vi "Exceldispatch.vi"() -> ()   [LabVIEW 2012]
uses:
  <vilib>/Utility/NIReport.llb/NI_report.lvclass
  Global1.vi
  <vilib>/addons/database/Connection.llb/DB Tools Open Connec (Path).vi
  <vilib>/addons/_office/excel.llb/Excel Get Data (str).vi
  <vilib>/Utility/NIReport.llb/Excel/NI_Excel.lvclass
  <vilib>/addons/_office/NI_ReportGenerationToolkit.lvlib
  <vilib>/addons/database/NI_Database_API.lvlib
panel:
  out "error out 4":errorcluster
  in  "start (0, 0)":cluster{"start row":i32, "start column":i32}
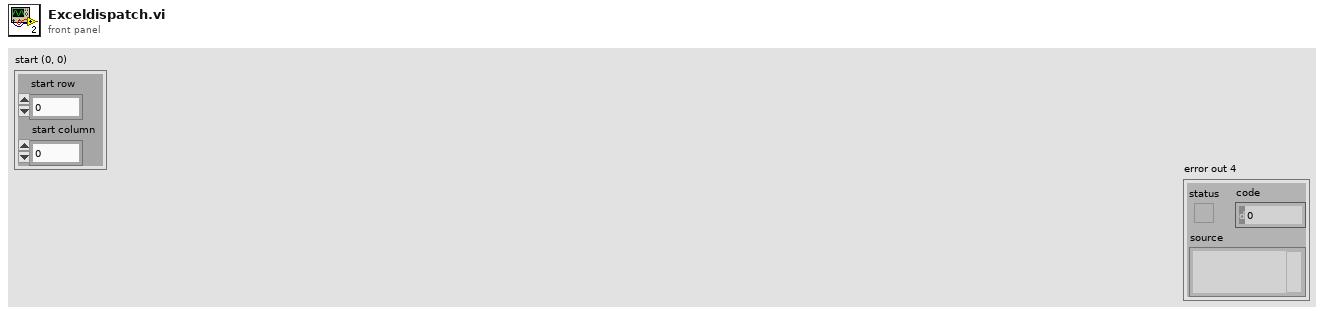
[diagram p1: front panel]
types:
  T1 = enum16{"Standard Report", "HTML", "Word", "Excel"}
  T2 = typedef "NI_Database_API.lvlib/Conn ObjectReference.ctl" = refnum<k1>
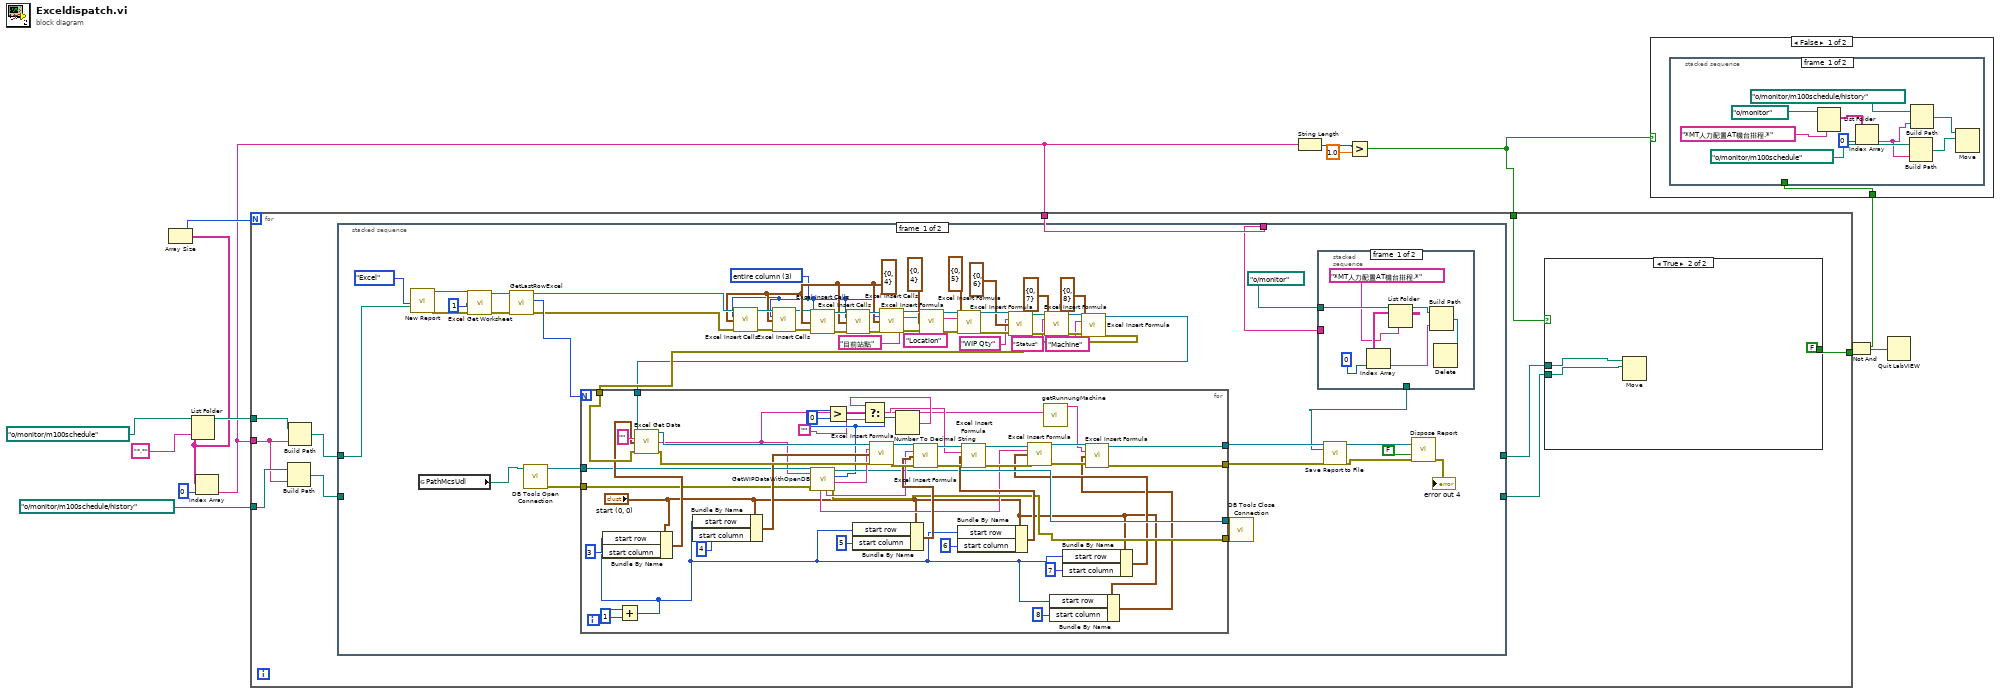
[diagram p0: block diagram]
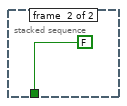
[diagram p2: hidden frame]
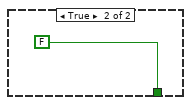
[diagram p3: hidden frame]
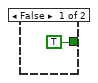
[diagram p4: hidden frame]
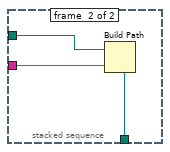
[diagram p5: hidden frame]
diagram:
  n1 = List Folder(path=path "o:/monitor/m100schedule", pattern="*.*") -> (path out=w10:path, filenames=w9:string[])  [unwired: 2 in, 2 out]
  n2 = Array Size(array=w9) -> (size(s)=w11:i32)
  n3 = Index Array(array=w9, index=0) -> (element=w3:string)
  n4 = String Length(string=w3) -> (length=w6:i32)
  n5 = Greater?(x=w6, y=1.0) -> (0:w2:bool)
  n6 = for {
    N: w11 -> [_]
    tunnel: w10 -> [w24]
    tunnel: w3 -> [w22]
    tunnel: path "o:/monitor/m100schedule/history" ("base path") -> [w23]
    tunnel: w2 -> [w17]
    tunnel: [w16] -> w4
    tunnel: w3 -> [w15]
    n7 = Build Path(base path=w23, name or relative path=w22) -> (appended path=w20:path)
    n8 = Build Path(base path=w24, name or relative path=w22) -> (appended path=w21:path)
    n9 = stacked-sequence {
      tunnel: w21 -> [w59 w141]
      tunnel: w20 -> [_ w142]
      tunnel: [_ w142] -> w18
      tunnel: [_ w141] -> w19
      tunnel: w15 -> [w30 _]
      frame #0 {
        w47 = cluster{"row":i32, "column":i32} {"row"=0, "column"=4} ("start (0, 0)")
        w44 = u16 3 items=["shift cells right", "shift cells down", "entire row", "entire column"] ("mode (entire row)")
        n10 = call <vilib>:"New Report.vi"("report type"=T1."Excel" ("Report Type"), "template (empty)"=w59) -> ("report out"=w83:refnum<class "NI_report.lvclass">, "error out"=w82:errorcluster)  [unwired: 12 in]
        n11 = global read "Global1.vi" "PathMcsUdl"() -> (w74:path)
        n12 = call <vilib>:"Excel Get Worksheet.vi"("report in"=w83, "worksheet index (0)"=1, "error in (no error)"=w82) -> ("report out"=w54:refnum<class "NI_report.lvclass">, "error out"=w53:errorcluster)  [unwired: 11 in]
        n13 = call "GetLastRowExcel.vi"("error in (no error)"=w53, "report in"=w54) -> ("error out"=w51:errorcluster, "row"=w52:i32, "report out"=w50:refnum<class "NI_report.lvclass">)  [unwired: 7 in]
        n14 = call-poly <vilib>:"DB Tools Open Connection.vi"("connection information"=w74) -> ("error out"=w72:errorcluster, "connection reference"=w73:T2)  [unwired: 7 in]
        n15 = call <vilib>:"Excel Insert Cells.vi"("report in"=w50, "mode (entire row)"=w44, "start (0, 0)"=w47, "error in (no error)"=w51) -> ("report out"=w49:refnum<class "NI_report.lvclass">, "error out"=w48:errorcluster)  [unwired: 10 in]
        n16 = call <vilib>:"Excel Insert Cells.vi"("report in"=w49, "mode (entire row)"=w44, "start (0, 0)"=w47, "error in (no error)"=w48) -> ("report out"=w46:refnum<class "NI_report.lvclass">, "error out"=w45:errorcluster)  [unwired: 10 in]
        n17 = call <vilib>:"Excel Insert Cells.vi"("report in"=w46, "mode (entire row)"=w44, "start (0, 0)"=w47, "error in (no error)"=w45) -> ("report out"=w80:refnum<class "NI_report.lvclass">, "error out"=w78:errorcluster)  [unwired: 10 in]
        n18 = call <vilib>:"Excel Insert Cells.vi"("report in"=w80, "mode (entire row)"=w44, "start (0, 0)"=w47, "error in (no error)"=w78) -> ("report out"=w79:refnum<class "NI_report.lvclass">, "error out"=w77:errorcluster)  [unwired: 10 in]
        n19 = call <vilib>:"Excel Insert Cells.vi"("report in"=w79, "mode (entire row)"=w44, "start (0, 0)"=w47, "error in (no error)"=w77) -> ("report out"=w71:refnum<class "NI_report.lvclass">, "error out"=w68:errorcluster)  [unwired: 10 in]
        n20 = call <vilib>:"Excel Insert Formula.vi"("report in"=w71, "formula"="目前站點", "start (0, 0)"=cluster{"row":i32, "column":i32} {"row"=0, "column"=4}, "error in (no error)"=w68) -> ("report out"=w70:refnum<class "NI_report.lvclass">, "error out"=w67:errorcluster)  [unwired: 10 in]
        n21 = call <vilib>:"Excel Insert Formula.vi"("report in"=w70, "formula"="Location", "start (0, 0)"=cluster{"row":i32, "column":i32} {"row"=0, "column"=5}, "error in (no error)"=w67) -> ("report out"=w69:refnum<class "NI_report.lvclass">, "error out"=w66:errorcluster)  [unwired: 10 in]
        n22 = call <vilib>:"Excel Insert Formula.vi"("report in"=w69, "formula"="WIP Qty", "start (0, 0)"=cluster{"row":i32, "column":i32} {"row"=0, "column"=6}, "error in (no error)"=w66) -> ("report out"=w43:refnum<class "NI_report.lvclass">, "error out"=w41:errorcluster)  [unwired: 10 in]
        n23 = call <vilib>:"Excel Insert Formula.vi"("report in"=w43, "formula"="Status", "start (0, 0)"=cluster{"row":i32, "column":i32} {"row"=0, "column"=7}, "error in (no error)"=w41) -> ("report out"=w42:refnum<class "NI_report.lvclass">, "error out"=w40:errorcluster)  [unwired: 10 in]
        n24 = call <vilib>:"Excel Insert Formula.vi"("report in"=w42, "formula"="Machine", "start (0, 0)"=cluster{"row":i32, "column":i32} {"row"=0, "column"=8}, "error in (no error)"=w40) -> ("report out"=w38:refnum<class "NI_report.lvclass">, "error out"=w39:errorcluster)  [unwired: 10 in]
        n25 = for {
          N: w52 -> [_]
          tunnel: w38 -> [w140]
          tunnel: w39 -> [w139]
          tunnel: [w103] -> w55
          tunnel: [w121] -> w76
          tunnel: [w120] -> w75
          tunnel: w73 -> [w119]
          tunnel: w72 -> [w118]
          tunnel: [w104] -> w35
          i -> [w111]
          n26 = Add(x=w111, y=1) -> (x+y=w100:i32)
          n27 = Bundle By Name(cluster="start (0, 0)", "start row"=w100, "start column"=3) -> (w134:cluster{"start row":i32, "start column":i32})
          n28 = call-poly <vilib>:"Excel Get Data.vi"("report in"=w140, "data type"="", "start (0, 0)"=w134, "error in (no error)"=w139) -> ("report out"=w137:refnum<class "NI_report.lvclass">, "data"=w95:string, "error out"=w136:errorcluster)  [unwired: 9 in]
          n29 = Bundle By Name(cluster="start (0, 0)", "start row"=w100, "start column"=4) -> (w132:cluster{"start row":i32, "start column":i32})
          n30 = call "GetWIPDataWithOpenDB.vi"("error in (no error)"=w118, "Lotno"=w95, "connection reference"=w119) -> ("error out"=w120:errorcluster, "step"=w123:string, "data"=w116:i32, "connection reference 2"=w121:T2, "location"=w122:string, "status"=w101:string)  [unwired: 3 in]
          n31 = Greater?(x=w116, y=0) -> (0:w114:bool)
          n32 = Bundle By Name(cluster="start (0, 0)", "start row"=w100, "start column"=5) -> (w124:cluster{"start row":i32, "start column":i32})
          n33 = call <vilib>:"Excel Insert Formula.vi"("report in"=w137, "formula"=w123, "start (0, 0)"=w132, "error in (no error)"=w136) -> ("report out"=w129:refnum<class "NI_report.lvclass">, "error out"=w126:errorcluster)  [unwired: 10 in]
          n34 = Number To Decimal String(number=w116) -> (decimal integer string=w115:string)  [unwired: 1 in]
          n35 = Select(t=w115, s=w114, f="") -> (s? t:f=w112:string)
          n36 = call <vilib>:"Excel Insert Formula.vi"("report in"=w129, "formula"=w122, "start (0, 0)"=w124, "error in (no error)"=w126) -> ("report out"=w128:refnum<class "NI_report.lvclass">, "error out"=w127:errorcluster)  [unwired: 10 in]
          n37 = Bundle By Name(cluster="start (0, 0)", "start row"=w100, "start column"=6) -> (w125:cluster{"start row":i32, "start column":i32})
          n38 = call <vilib>:"Excel Insert Formula.vi"("report in"=w128, "formula"=w112, "start (0, 0)"=w125, "error in (no error)"=w127) -> ("report out"=w108:refnum<class "NI_report.lvclass">, "error out"=w107:errorcluster)  [unwired: 10 in]
          n39 = call "getRunnungMachine.vi"("rc_no"=w95) -> ("machine"=w96:string)  [unwired: 9 in, 1 out]
          n40 = Bundle By Name(cluster="start (0, 0)", "start row"=w100, "start column"=8) -> (w98:cluster{"start row":i32, "start column":i32})
          n41 = Bundle By Name(cluster="start (0, 0)", "start row"=w100, "start column"=7) -> (w102:cluster{"start row":i32, "start column":i32})
          n42 = call <vilib>:"Excel Insert Formula.vi"("report in"=w108, "formula"=w101, "start (0, 0)"=w102, "error in (no error)"=w107) -> ("report out"=w106:refnum<class "NI_report.lvclass">, "error out"=w105:errorcluster)  [unwired: 10 in]
          n43 = call <vilib>:"Excel Insert Formula.vi"("report in"=w106, "formula"=w96, "start (0, 0)"=w98, "error in (no error)"=w105) -> ("report out"=w104:refnum<class "NI_report.lvclass">, "error out"=w103:errorcluster)  [unwired: 10 in]
        }
        n44 = call <vilib>:"DB Tools Close Connection.vi"("error in (no error)"=w75, "connection reference"=w76) -> ()  [unwired: 5 in, 1 out]
        n45 = stacked-sequence {
          tunnel: path "o:/monitor" ("base path") -> [w87 w94]
          tunnel: w30 -> [_ w93]
          tunnel: [_ w92] -> w29
          frame #0 {
            n46 = List Folder(path=w87, pattern="*MT人力配置AT機台排程.*") -> (path out=w89:path, filenames=w91:string[])  [unwired: 2 in, 2 out]
            n47 = Index Array(array=w91, index=0) -> (element=w88:string)
            n48 = Build Path(base path=w89, name or relative path=w88) -> (appended path=w85:path)
            n49 = Delete(path (use dialog)=w85) -> ()  [unwired: 4 in, 3 out]
          }
          frame #1 {
            n50 = Build Path(base path=w94, name or relative path=w93) -> (appended path=w92:path)
          }
        }
        n51 = call-dynamic "Save Report to File.vi"("report in"=w35, "report file path"=w29, "error in (no error)"=w55) -> ("report out"=w34:refnum<class "NI_report.lvclass">, "error out"=w56:errorcluster)  [unwired: 11 in]
        n52 = call-dynamic "Dispose Report.vi"("report in"=w34, "save changes? (F)"=FALSE, "error in (no error)"=w56) -> ("error out"=→"error out 4":errorcluster)  [unwired: 12 in]
      }
      frame #1 {
      }
    }
    n53 = case shown="True" w17 {
      tunnel: [TRUE FALSE] -> w16
      tunnel: w19 -> [_ w27]
      tunnel: w18 -> [_ w26]
      frame False {
      }
      frame True {
        n54 = Move(source path=w27, 10:w26) -> ()  [unwired: 3 in, 3 out]
      }
    }
  }
  n55 = case shown="False" w2 {
    tunnel: [w143 FALSE] -> w1
    frame False {
      n56 = stacked-sequence {
        tunnel: [_ FALSE] -> w143
        frame #0 {
          n57 = List Folder(path=path "o:/monitor", pattern="*MT人力配置AT機台排程.*") -> (filenames=w151:string[])  [unwired: 2 in, 3 out]
          n58 = Index Array(array=w151, index=0) -> (element=w145:string)
          n59 = Build Path(base path=path "o:/monitor/m100schedule", name or relative path=w145) -> (appended path=w147:path)
          n60 = Build Path(base path=path "o:/monitor/m100schedule/history", name or relative path=w145) -> (appended path=w149:path)
          n61 = Move(source path=w149, 10:w147) -> ()  [unwired: 3 in, 3 out]
        }
        frame #1 {
        }
      }
    }
    frame True {
    }
  }
  n62 = Not And(1:w4, 2:w1) -> (0:w5:bool)
  n63 = Quit LabVIEW(quit? (T)=w5) -> ()
